vi "Agilent SNA Send Cancel Pass Through Command.vi"(6 "SCPI? (F)":bool, 7 "Agilent SNA & SWP":T1, 8 "error in (no error)":errorcluster, 11 "VISA Resource Names":T2) -> (0 "error out":errorcluster, 3 "dup VISA Resource Names":T2)   [LabVIEW 2011]
doc: "This VI for the HP8753B Network Analyzers reads the stimulus values. Except when performing log sweeps and freq list sweeps, this VI uses the start and stop values and the number of points to calcuate the stimulus values."
uses:
  TypeDefs/Agilent SNA VISA.ctl
  TypeDefs/Agilent SNA Instrument Info.ctl
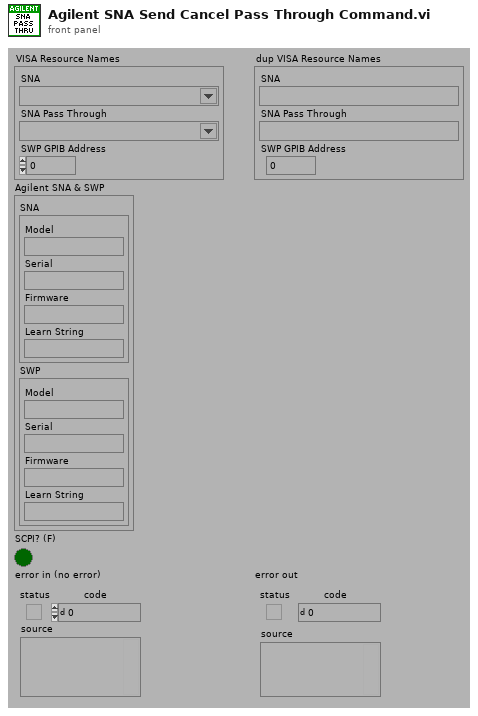
[diagram p1: front panel]
types:
  T1 = typedef "Agilent SNA Instrument Info.ctl" = cluster{"SNA":cluster{"Model":string, "Serial":string, "Firmware":string, "Learn String":string}, "SWP":cluster{"Model":string, "Serial":string, "Firmware":string, "Learn String":string}}
  T2 = typedef "Agilent SNA VISA.ctl" = cluster{"SNA":refnum<visa-resource-name>, "SNA Pass Through":refnum<visa-resource-name>, "SWP GPIB Address":i32}
  T3 = typedef "Agilent SNA SWP Model.ctl" = enum16{"Not Supported", "836XXX", "8375XX", "E82X7D"}
  T4 = typedef "Agilent SNA Model.ctl" = enum16{"Not Supported", "8757X"}
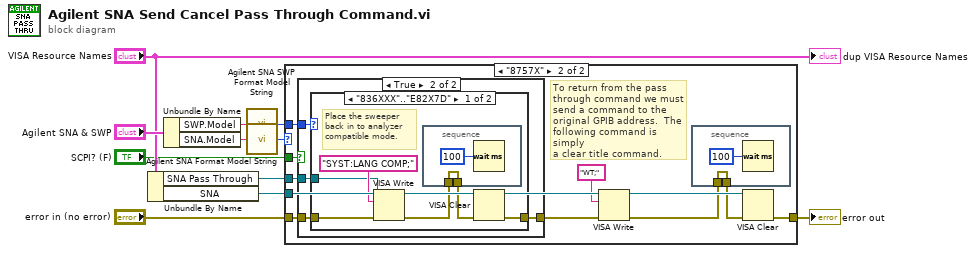
[diagram p0: block diagram]
diagram:
  n1 = Unbundle By Name("VISA Resource Names") -> ("SNA Pass Through"=w2:refnum<visa-resource-name>, "SNA"=w5:refnum<visa-resource-name>)
  n2 = Unbundle By Name("Agilent SNA & SWP") -> ("SWP.Model"=w4:string, "SNA.Model"=w8:string)
  n3 = call "Agilent SNA SWP Format Model String.vi"("Model String"=w4) -> ("Model"=w3:T3)
  n4 = call "Agilent SNA Format Model String.vi"("Model String"=w8) -> ("Model"=w7:T4)
  n5 = case shown="\"8757X\"" w7 {
    tunnel: [w12 w15] -> w11
    tunnel: "error in (no error)" -> [w12 w21]
    tunnel: w5 -> [_ w23]
    tunnel: w3 -> [_ w18]
    tunnel: w2 -> [_ w19]
    tunnel: "SCPI? (F)" -> [_ w17]
    frame "Not Supported" {
    }
    frame "8757X" {
      # "To return from the pass\nthrough command we must\nsend a command to the\noriginal GPIB address.  The\nfollowing command is simply\na clear title command."
      n6 = case shown="True" w17 {
        tunnel: w21 -> [w26 w30]
        tunnel: [w26 w29] -> w20
        tunnel: w19 -> [_ w28]
        tunnel: w18 -> [_ w27]
        frame False {
          # "The analyzer was not\nput into SCPI mode, so\nthere is no need to set\nit back."
        }
        frame True {
          n7 = case shown="\"836XXX\"..\"E82X7D\"" w27 {
            tunnel: w30 -> [w37 w40]
            tunnel: [w33 w40] -> w29
            tunnel: w28 -> [w35 _]
            frame "836XXX".."E82X7D" {
              # "Place the sweeper\nback in to analyzer\ncompatible mode."
              n8 = VISA Write(VISA resource name=w35, write buffer="SYST:LANG COMP;" ("format string"), error in (no error)=w37) -> (VISA resource name out=w34:refnum<visa-resource-name>, error out=w32:errorcluster)  [unwired: 1 out]
              n9 = stacked-sequence {
                tunnel: w32 -> [w38]
                tunnel: [w38] -> w31
                frame #0 {
                  n10 = Wait (ms)(milliseconds to wait=u32 100) -> ()  [unwired: 1 out]
                }
              }
              n11 = VISA Clear(VISA resource name=w34, error in (no error)=w31) -> (error out=w33:errorcluster)  [unwired: 1 out]
            }
            frame "Not Supported" {
            }
          }
        }
      }
      n12 = VISA Write(VISA resource name=w23, write buffer="WT;", error in (no error)=w20) -> (VISA resource name out=w16:refnum<visa-resource-name>, error out=w14:errorcluster)  [unwired: 1 out]
      n13 = stacked-sequence {
        tunnel: w14 -> [w24]
        tunnel: [w24] -> w13
        frame #0 {
          n14 = Wait (ms)(milliseconds to wait=u32 100) -> ()  [unwired: 1 out]
        }
      }
      n15 = VISA Clear(VISA resource name=w16, error in (no error)=w13) -> (error out=w15:errorcluster)  [unwired: 1 out]
    }
  }
  "error out" <- w11
  "dup VISA Resource Names" <- "VISA Resource Names"
